vi "To Device Identity.vi"(8 "error in":errorcluster, 10 "System Identifier":string="IDN:OXFORD INSTRUMENTS:MERCURY ITC:123456:SW_VERSION") -> (0 "error out":errorcluster, 1 "Instrument Valid":bool, 2 "S/W Version":string, 3 "Serial Number":string)   [LabVIEW 2015, in "Mercury iXX.lvlib"]
uses:
  Mercury iXX.lvlib
panel:
  # "IDN:OXFORD INSTRUMENTS:MERCURY ITC:123456:SW_VERSION"
  # "IDN:OXFORD INSTRUMENTS:MERCURY IPS:123457:SW_VERSION"
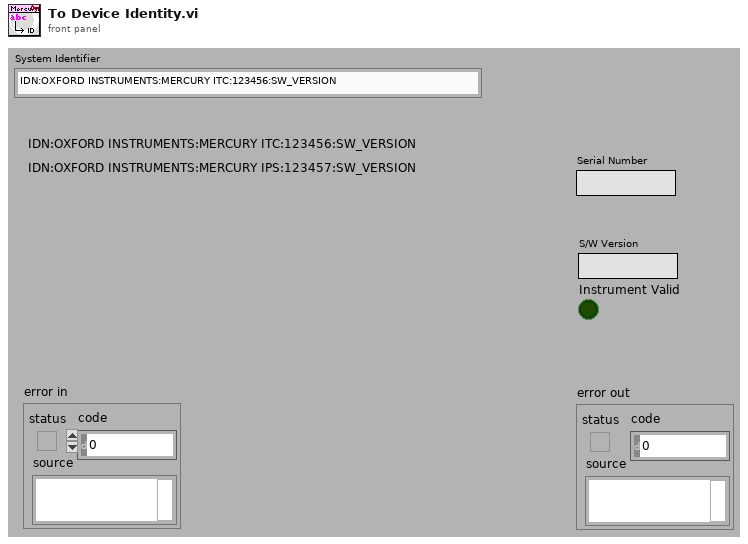
[diagram p1: front panel]
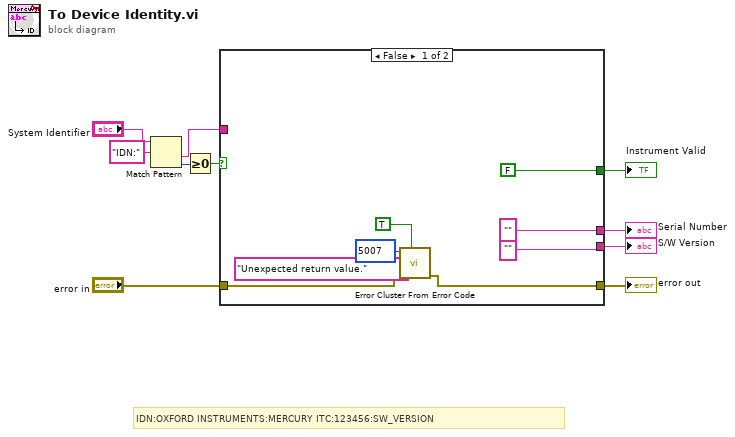
[diagram p0: block diagram]
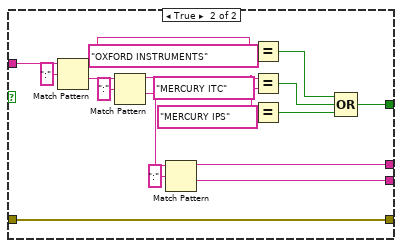
[diagram p2: hidden frame]
diagram:
  # "IDN:OXFORD INSTRUMENTS:MERCURY ITC:123456:SW_VERSION"
  n1 = Match Pattern(string="System Identifier", regular expression="IDN:") -> (after substring=w4:string, offset past match=w10:i32)  [unwired: 3 out]
  n2 = Greater Or Equal To 0?(x=w10) -> (x >= 0?=w8:bool)
  n3 = case shown="False" w8 {
    tunnel: w4 -> [_ w36]
    tunnel: [w17 w34] -> w7
    tunnel: "error in" -> [w12 w34]
    tunnel: [FALSE w21] -> w3
    tunnel: ["" ("System Identifier") w20] -> w2
    tunnel: ["" ("System Identifier") w19] -> w1
    frame False {
      n4 = call <vilib>:"Error Cluster From Error Code.vi"("show call chain? (False)"=TRUE, "error in (no error)"=w12, "error message (\"\")"="Unexpected return value." ("error message (\"\")"), "error code (0)"=5007) -> ("error out"=w17:errorcluster)  [unwired: 5 out]
    }
    frame True {
      n5 = Match Pattern(string=w36, regular expression=":") -> (before substring=w30:string, after substring=w33:string)  [unwired: 3 out]
      n6 = Match Pattern(string=w33, regular expression=":") -> (before substring=w26:string, after substring=w31:string)  [unwired: 3 out]
      n7 = Match Pattern(string=w31, regular expression=":") -> (before substring=w20:string, after substring=w19:string)  [unwired: 3 out]
      n8 = Equal?(x=w30, y="OXFORD INSTRUMENTS") -> (x = y?=w23:bool)
      n9 = Equal?(x=w26, y="MERCURY ITC") -> (x = y?=w25:bool)
      n10 = Equal?(x=w26, y="MERCURY IPS") -> (x = y?=w24:bool)
      n11 = Compound Arithmetic op=OR(w23, w25, w24) -> (w21:bool)
    }
  }
  "error out" <- w7
  "Instrument Valid" <- w3
  "Serial Number" <- w2
  "S/W Version" <- w1
